vi "Open.vi"(8 "error in (no error)":errorcluster, 10 "VISA resource name":refnum<visa-resource-name>="COM3", 11 "ThermPID in":refnum<class "ThermPID.lvclass">) -> (0 "error out":errorcluster, 3 "ThermPID out":refnum<class "ThermPID.lvclass">)   [LabVIEW 2023, in "ThermPID.lvclass"]
uses:
  ThermPID.lvclass
  ThermPID.lvclass/ThermPID.ctl
  <vilib>/NI/Modbus Library/API/Wrapper/Create Serial Master.vi
  <vilib>/NI/Modbus Library/API/Wrapper/API Main.lvlib
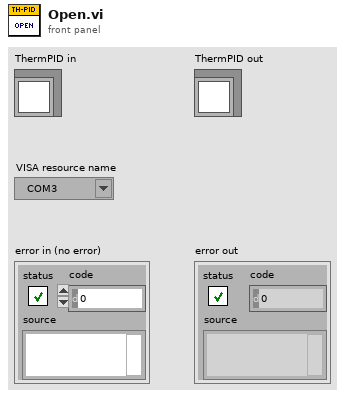
[diagram p1: front panel]
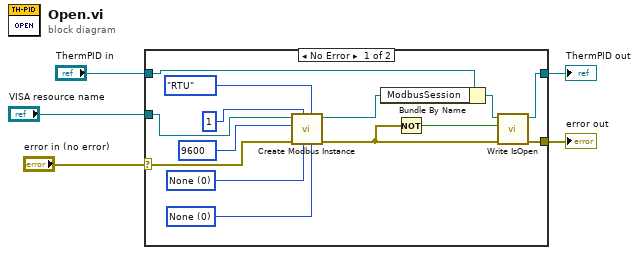
[diagram p0: block diagram]
diagram:
  n1 = case shown="No Error" "error in (no error)" {
    selector: "error in (no error)" -> [w12 w21]
    tunnel: [w6 w21] -> w4
    tunnel: [w9 w20] -> w2
    tunnel: "ThermPID in" -> [w19 w20]
    tunnel: "VISA resource name" -> [w13 _]
    frame No Error {
      w18 = u16 0 items=["None", "XON/XOFF", "RTS/CTS", "XON/XOFF & RTS/CTS", "DTR/DSR", "XON/XOFF & DTR/DSR"] ("flow control")
      w17 = u16 0 items=["None", "Odd", "Even", "Mark", "Space"] ("parity (even)")
      n2 = call-poly <vilib>:"Create Modbus Instance.vi"("flow control (none)"=w18, "serial type"=enum16{"RTU", "ASCII"}."RTU", "parity (even)"=w17, "unit ID"=u8 1, "error in"=w12, "baud rate"=u32 9600, "VISA resource name"=w13) -> ("error out"=w7:errorcluster, "serial master instance"=w11:refnum<class "Modbus Master.lvclass">)  [unwired: 3 in]
      n3 = Bundle By Name(cluster=w19, "ModbusSession"=w11) -> (w10:refnum<class "ThermPID.lvclass">)
      n4 = Not(x=w7) -> (.not. x?=w8:bool)
      n5 = call-dynamic "Write IsOpen.vi"("error in (no error)"=w7, "IsOpen"=w8, "PIDController in"=w10) -> ("error out"=w6:errorcluster, "PIDController out"=w9:refnum<class "ThermPID.lvclass">)  [unwired: 7 in]
    }
    frame Error {
    }
  }
  "error out" <- w4
  "ThermPID out" <- w2
